vi "Enqueue.vi"(8 "error in (no error)":errorcluster, 10 "Data":variant, 11 "State":T1) -> (0 "error out":errorcluster)   [LabVIEW 2018, in "User Console.lvlib"]
doc: "Enqueues elements to the module queue."
uses:
  User Console.lvlib
  ctl/Module State--enum.ctl
  Module Queue Actions.ctl
  ctl/Module Message--cluster.ctl
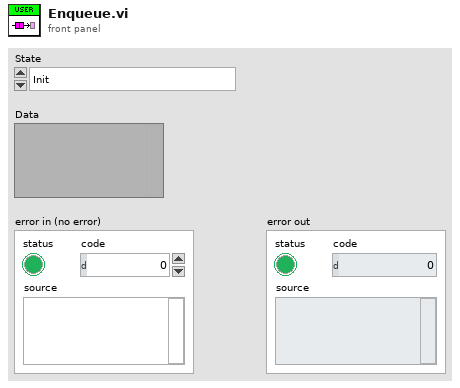
[diagram p1: front panel]
types:
  T1 = typedef "User Console.lvlib/Module State--enum.ctl" = enum16{"Init", "Error", "Idle", "Close", "Transaction Button Pressed: Which?", "Balance Inquiry Pressed", "Desposit Pressed", "Withdrawal Pressed", "Fast Cash Pressed", "New Transaction Pressed", "Terminate Session Pressed", "Card Reader Pressed", "Keypad Button Pressed", "Update Keypad Screen", "Enable/disable controls", "Card reader: On?"}
  T2 = typedef "User Console.lvlib/Module Message--cluster.ctl" = cluster{"State":T1, "Data":variant}
  T3 = typedef "User Console.lvlib/Module Queue Actions.ctl" = enum16{"Create", "Get", "Destroy"}
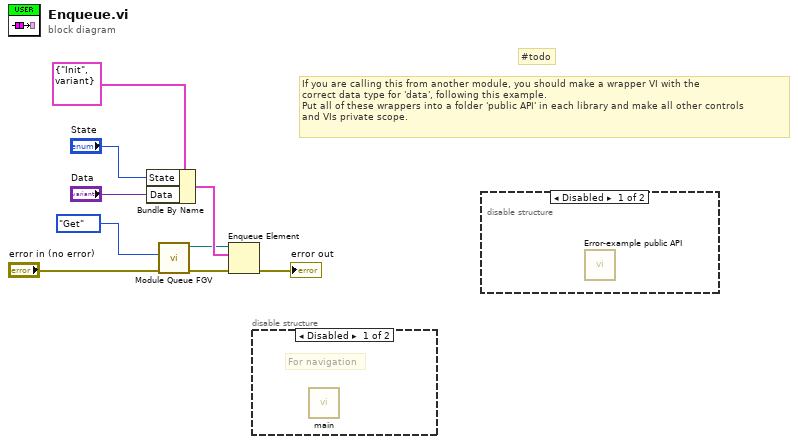
[diagram p0: block diagram]
diagram:
  # "If you are calling this from another module, you should make a wrapper VI with the\ncorrect data type for 'data', following this example.\nPut all of these wrappers into a folder 'public API' in each library and make all other controls \nand VIs private scope."
  # "#todo"
  n1 = Bundle By Name(cluster=T2 {"State"=enum."Init", "Data"=variant} ("element"), "State"="State", "Data"="Data") -> (w7:T2)
  n2 = call "Module Queue FGV.vi"("Error in"="error in (no error)", "Module Queue Actions"=Module_Queue_Actions."Get") -> ("error out"=w3:errorcluster, "Queue out"=w2:refnum<queue>)  [unwired: 8 in]
  n3 = Enqueue Element(queue=w2, element=w7, error in (no error)=w3) -> (error out=→"error out":errorcluster)  [unwired: 1 in, 2 out]
  n4 = disable-structure shown="Disabled" {
    frame Disabled {
      # "For navigation"
      n5 = call "main.vi"() -> ()  [unwired: 11 in, 1 out]
    }
    frame Enabled {
    }
  }
  n6 = disable-structure shown="Disabled" {
    frame Disabled {
      n7 = call "Error-example public API.vi"() -> ()  [unwired: 11 in, 1 out]
    }
    frame Enabled {
    }
  }
